vi "Get SMO Port.vi"(8 "error in (no error)":errorcluster, 11 "Inst.Framework-TemplateInstrument in":refnum<class "Inst.Framework-Template.lvclass">) -> (0 "error out":errorcluster, 2 "Port":u16, 3 "Inst.Framework-TemplateInstrument out":refnum<class "Inst.Framework-Template.lvclass">)   [LabVIEW 2019, in "Inst.Framework-Template.lvclass"]
uses:
  Inst.Framework-Template.lvclass
  <userlib>/LevyLab/Instrument Framework/Instrument Types/VSource/Instrument.VSource.lvclass
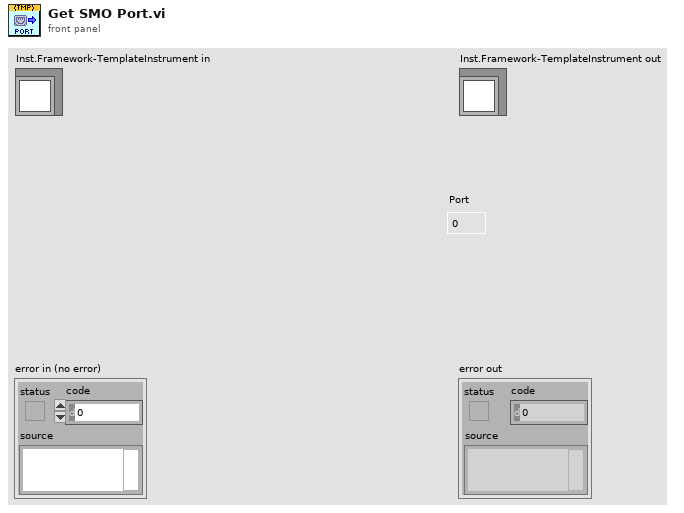
[diagram p1: front panel]
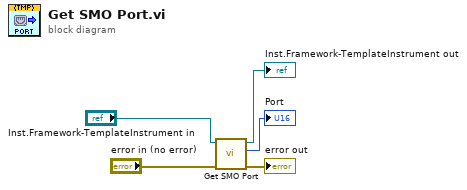
[diagram p0: block diagram]
diagram:
  n1 = call-parent "Get SMO Port.vi"("error in (no error)"="error in (no error)", "Instrument in"="Inst.Framework-TemplateInstrument in") -> ("error out"=→"error out":errorcluster, "Port"=→"Port":u16, "Instrument out"=→"Inst.Framework-TemplateInstrument out":refnum<class "Inst.Framework-Template.lvclass">)  [unwired: 7 in]
